vi "setExternSensor.vi"(8 "error in (no error)":errorcluster, 10 "ExternalSensorStatus":T1, 11 "CoolerControler in":refnum<class "CoolerControler.lvclass">) -> (0 "error out":errorcluster, 2 "ExternalSensorStatus out":T1, 3 "CoolerControler out":refnum<class "CoolerControler.lvclass">)   [LabVIEW 2016, in "CoolerControler.lvclass"]
uses:
  CoolerControler.lvclass
  typedefs/ExternalSensorStatus.ctl
  SerialCommand/CoolerSerialCommand.lvclass
  typedefs/dataUnit.ctl
  typedefs/CoolerCommands.ctl
  typedefs/CoolerId.ctl
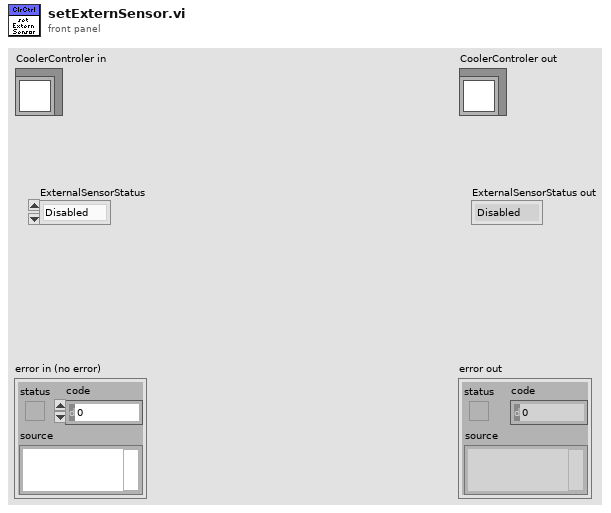
[diagram p1: front panel]
types:
  T1 = typedef "ExternalSensorStatus.ctl" = enum16{"Disabled", "Enabled"}
  T2 = typedef "CoolerId.ctl" = u16
  T3 = typedef "CoolerCommands.ctl" = enum16{"None", "SetExternSensorStatus", "SetChillerStatus", "SetControlSensor", "SetControlTemperature", "SetHighSupplyTempWarning", "SetLowSupplyTemperatureWarning", "SetHighAmbientTemperatureWarning", "SetLowAmbienTemperatureWarning", "SetLowProcessFlowWarning", "SetHighSupplyTemperatureAlarm", "SetLowSupplyTemperatureAlarm", "SetHighAmbientTemperatureAlarm", "SetLowAmbientTemperatureAlarm", "SetLowProcessFlowAlarm"}
  T4 = typedef "dataUnit.ctl" = enum16{"temperature", "flow", "current", "PID", "fanSpeed", "time", "PWM", "TEDriveLevel", "Number"}
  T5 = typedef "response.ctl" = cluster{"deviceId":string, "commandNumber":string, "errorActive":bool, "commandName":string, "responseData":string, "checkSum":string}
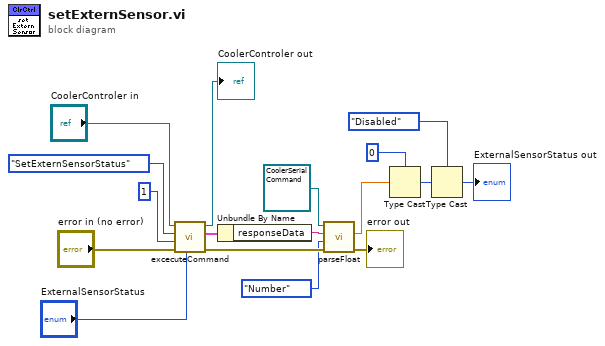
[diagram p0: block diagram]
diagram:
  n1 = call "excecuteCommand.vi"("inputValue"="ExternalSensorStatus", "error in (no error)"="error in (no error)", "id"=T2 1, "CoolerCommand"=CoolerCommands."SetExternSensorStatus", "CoolerControler in"="CoolerControler in") -> ("error out"=w16:errorcluster, "response out"=w15:T5, "CoolerControler out"=→"CoolerControler out":refnum<class "CoolerControler.lvclass">)  [unwired: 4 in]
  n2 = Unbundle By Name(w15) -> ("responseData"=w13:string)
  n3 = call "parseFloat.vi"("error in (no error)"=w16, "unit"=dataUnit."Number", "commandData"=w13, "CoolerSerialCommand in"=refnum<class "CoolerSerialCommand.lvclass"> refnum) -> ("error out"=→"error out":errorcluster, "value"=w9:sgl)  [unwired: 4 in, 2 out]
  n4 = Type Cast(type=u16 0, x=w9) -> (*(type *) &x=w11:u16)
  n5 = Type Cast(type=ExternalSensorStatus."Disabled" ("ExternalSensorStatus out"), x=w11) -> (*(type *) &x=→"ExternalSensorStatus out":T1)
